vi "tm485_lightsheet.vi"() -> ()   [LabVIEW 2011]
panel:
  in  "Input Trigger Polarity":u32(ring)=1 items=["NEGATIVE"=1, "POSITIVE"=2]
  in  "Input Trigger Mode":u32(ring)=1 items=["INTERNAL"=1, "EXTERNAL EDGE"=2, "EXTERNAL LEVEL"=4, "SOFTWARE"=32, "FAST REPETITION"=64, "TDI"=128, "START"=512, "SYNC READOUT"=1024]
  in  "Internal Line Interval":dbl=9.74436e-06
  in  "Output Trigger Period":dbl=1e-05
  in  "Output Trigger Polarity":u32(ring)=1 items=["NEGATIVE"=1, "POSITIVE"=2]
  in  "Output Trigger Mode":u32(ring)=3 items=["LOW"=1, "GLOBAL EXPOSURE"=2, "PROGRAMMABLE"=3, "TRIGGER READY"=4, "HIGH"=5]
  in  "Readout Direction":u32(ring)=1 items=["FORWARD"=1, "BACKWARD"=2]
  in  "Pre Hsync Count":u32
  out "Image":u16[][](graph)
  out "Frames Per Second":dbl
  in  "Quit":bool
  out "Error Out":errorcluster {"code" format="%.0x"}
  # "This is just a simple example\nof how to setup a camera for\na Lightsheet application with\na Flash4.0 V2"
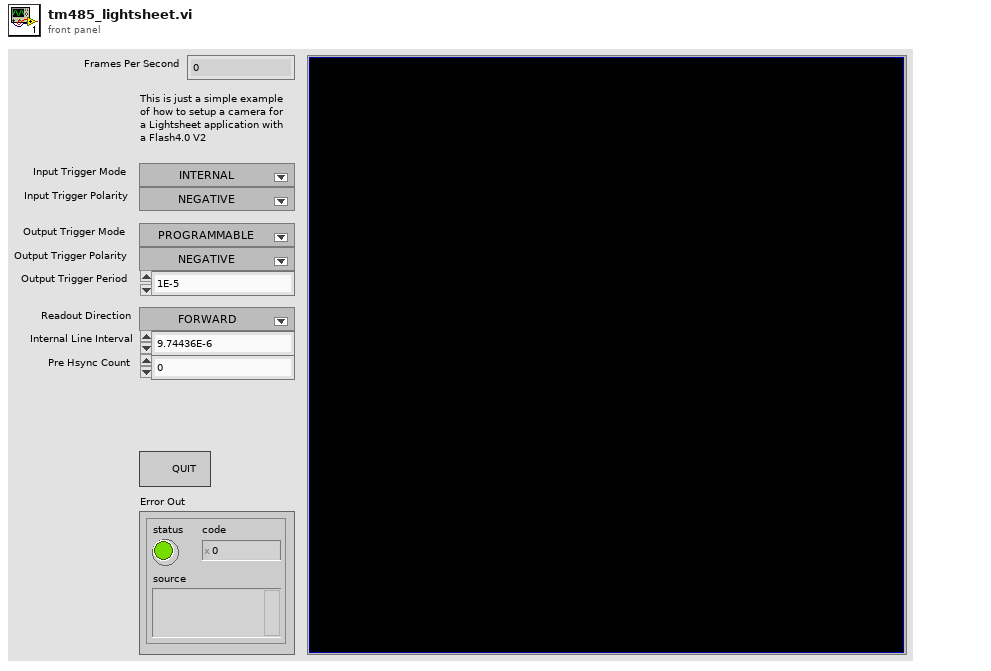
[diagram p1: front panel]
types:
  T1 = cluster{"Input Trigger Mode":u32, "Input Trigger Polarity":u32, "Times":u32, "Delay":dbl}
  T2 = cluster{"Output Trigger Mode":u32, "Output Trigger Polarity":u32}
  T3 = cluster{"Output Trigger Period":dbl, "Delay":dbl, "Source":u32}
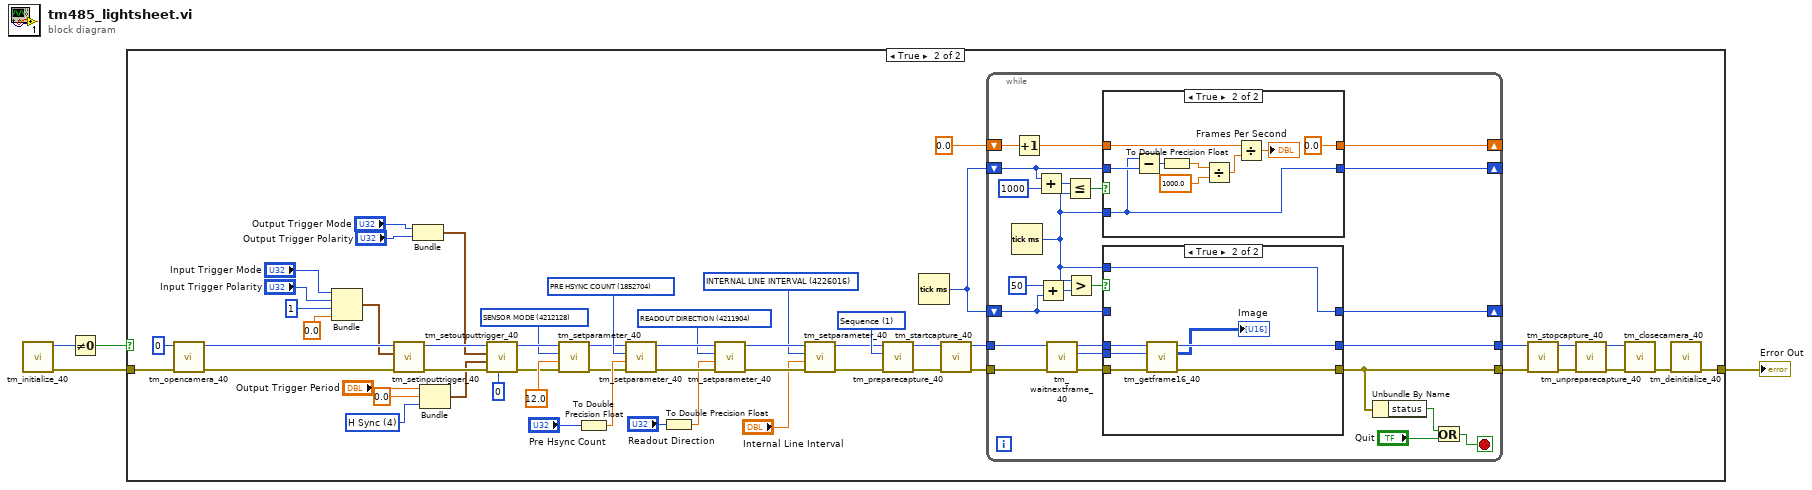
[diagram p0: block diagram]
diagram:
  n1 = call <userlib>:"tm_initialize_40.vi"() -> ("error out"=w1:errorcluster, "Number Of Cameras"=w2:u32)  [unwired: 8 in, 2 out]
  n2 = Not Equal To 0?(x=w2) -> (x != 0?=w4:bool)
  n3 = case shown="True" w4 {
    tunnel: w1 -> [w5 w59]
    tunnel: [w5 w56] -> w3
    frame False {
    }
    frame True {
      w8 = u32 4 items=["Exposure"=1, "Readout End"=2, "V Sync"=3, "H Sync"=4, "Trigger"=6] ("Source")
      w20 = u32 4226016 items=["SENSOR MODE"=4212128, "CCD MODE"=4212384, "READOUT MODE"=4211872, "ACTIVE VIEW INDEX"=4343136, "BITS PER CHANNEL"=4342976, "IMAGE PIXEL TYPE"=4343296, "BINNING"=4215968, "EXPOSURE TIME"=2049184, "CONTRAST GAIN"=3163312, "CONTRAST OFFSET"=3163328, "LIGHT MODE"=2114720, "SENSITIVITY"=2114992, "PHOTON IMAGING MODE"=2115200, "HIGH DYNAMIC RANGE MODE"=3163360, "WHITE BALANCE"=3163568, "TEMPERATURE"=2115232, "TEMPERATURE TARGET"=2115264, "SENSOR COOLER FAN"=2115296, "LINEBUNDLE HEIGHT"=4212192, "MECHANICAL SHUTTER"=2115488, "BACK FOCUS POSITION"=8422304, "TRIGGER CONNECTOR"=1066432, "TRIGGER SOURCE"=1066144, "OUTPUT TRIGGER SOURCE"=1852576, "TRIGGER GLOBAL EXPOSURE"=2049680, "FIRST TRIGGER BEHAVIOR"=2049696, "CHANNEL SYNC"=1852352, "READOUT DIRECTION"=4211904, "PRE HSYNC COUNT"=1852704, "INTERNAL LINE SPEED"=4226000, "INTERNAL LINE INTERVAL"=4226016] ("Parameter")
      w26 = u32 4212128 items=["SENSOR MODE"=4212128, "CCD MODE"=4212384, "READOUT MODE"=4211872, "ACTIVE VIEW INDEX"=4343136, "BITS PER CHANNEL"=4342976, "IMAGE PIXEL TYPE"=4343296, "BINNING"=4215968, "EXPOSURE TIME"=2049184, "CONTRAST GAIN"=3163312, "CONTRAST OFFSET"=3163328, "LIGHT MODE"=2114720, "SENSITIVITY"=2114992, "PHOTON IMAGING MODE"=2115200, "HIGH DYNAMIC RANGE MODE"=3163360, "WHITE BALANCE"=3163568, "TEMPERATURE"=2115232, "TEMPERATURE TARGET"=2115264, "SENSOR COOLER FAN"=2115296, "LINEBUNDLE HEIGHT"=4212192, "MECHANICAL SHUTTER"=2115488, "BACK FOCUS POSITION"=8422304, "TRIGGER CONNECTOR"=1066432, "TRIGGER SOURCE"=1066144, "OUTPUT TRIGGER SOURCE"=1852576, "TRIGGER GLOBAL EXPOSURE"=2049680, "FIRST TRIGGER BEHAVIOR"=2049696, "CHANNEL SYNC"=1852352, "READOUT DIRECTION"=4211904, "PRE HSYNC COUNT"=1852704, "INTERNAL LINE SPEED"=4191408, "INTERNAL LINE INTERVAL"=4191424] ("Parameter")
      w27 = u32 1852704 items=["SENSOR MODE"=4212128, "CCD MODE"=4212384, "READOUT MODE"=4211872, "ACTIVE VIEW INDEX"=4343136, "BITS PER CHANNEL"=4342976, "IMAGE PIXEL TYPE"=4343296, "BINNING"=4215968, "EXPOSURE TIME"=2049184, "CONTRAST GAIN"=3163312, "CONTRAST OFFSET"=3163328, "LIGHT MODE"=2114720, "SENSITIVITY"=2114992, "PHOTON IMAGING MODE"=2115200, "HIGH DYNAMIC RANGE MODE"=3163360, "WHITE BALANCE"=3163568, "TEMPERATURE"=2115232, "TEMPERATURE TARGET"=2115264, "SENSOR COOLER FAN"=2115296, "LINEBUNDLE HEIGHT"=4212192, "MECHANICAL SHUTTER"=2115488, "BACK FOCUS POSITION"=8422304, "TRIGGER CONNECTOR"=1066432, "TRIGGER SOURCE"=1066144, "OUTPUT TRIGGER SOURCE"=1852576, "TRIGGER GLOBAL EXPOSURE"=2049680, "FIRST TRIGGER BEHAVIOR"=2049696, "CHANNEL SYNC"=1852352, "READOUT DIRECTION"=4211904, "PRE HSYNC COUNT"=1852704, "INTERNAL LINE SPEED"=4191408, "INTERNAL LINE INTERVAL"=4191424] ("Parameter")
      w28 = u32 4211904 items=["SENSOR MODE"=4212128, "CCD MODE"=4212384, "READOUT MODE"=4211872, "ACTIVE VIEW INDEX"=4343136, "BITS PER CHANNEL"=4342976, "IMAGE PIXEL TYPE"=4343296, "BINNING"=4215968, "EXPOSURE TIME"=2049184, "CONTRAST GAIN"=3163312, "CONTRAST OFFSET"=3163328, "LIGHT MODE"=2114720, "SENSITIVITY"=2114992, "PHOTON IMAGING MODE"=2115200, "HIGH DYNAMIC RANGE MODE"=3163360, "WHITE BALANCE"=3163568, "TEMPERATURE"=2115232, "TEMPERATURE TARGET"=2115264, "SENSOR COOLER FAN"=2115296, "LINEBUNDLE HEIGHT"=4212192, "MECHANICAL SHUTTER"=2115488, "BACK FOCUS POSITION"=8422304, "TRIGGER CONNECTOR"=1066432, "TRIGGER SOURCE"=1066144, "OUTPUT TRIGGER SOURCE"=1852576, "TRIGGER GLOBAL EXPOSURE"=2049680, "FIRST TRIGGER BEHAVIOR"=2049696, "CHANNEL SYNC"=1852352, "READOUT DIRECTION"=4211904, "PRE HSYNC COUNT"=1852704, "INTERNAL LINE SPEED"=4191408, "INTERNAL LINE INTERVAL"=4191424] ("Parameter")
      w47 = 1 items=["Snap", "Sequence"] ("Capture mode")
      n4 = call <userlib>:"tm_opencamera_40.vi"("error in (no error)"=w59, "Camera Index"=u32 0) -> ("error out"=w31:errorcluster, "Handle out"=w32:u32)  [unwired: 7 in, 1 out]
      n5 = Bundle("Input Trigger Mode"="Input Trigger Mode", "Input Trigger Polarity"="Input Trigger Polarity", "Times"=u32 1, "Delay"=0.0) -> (w19:T1)  [unwired: 1 in]
      n6 = call <userlib>:"tm_setinputtrigger_40.vi"("error in (no error)"=w31, "Parameters"=w19, "Handle in"=w32) -> ("error out"=w34:errorcluster, "Handle out"=w33:u32)  [unwired: 7 in]
      n7 = Bundle("Output Trigger Mode"="Output Trigger Mode", "Output Trigger Polarity"="Output Trigger Polarity") -> (w12:T2)  [unwired: 1 in]
      n8 = Bundle("Output Trigger Period"="Output Trigger Period", "Delay"=0.0, "Source"=w8) -> (w11:T3)  [unwired: 1 in]
      n9 = call <userlib>:"tm_setoutputtrigger_40.vi"("Port"=0 ("Index"), "error in (no error)"=w34, "Programmable Options"=w11, "Type"=w12, "Handle in"=w33) -> ("error out"=w29:errorcluster, "Handle out"=w30:u32)  [unwired: 5 in]
      n10 = call <userlib>:"tm_setparameter_40.vi"("error in (no error)"=w29, "Value in"=12.0, "Parameter"=w26, "Handle in"=w30) -> ("error out"=w6:errorcluster, "Handle out"=w7:u32)  [unwired: 6 in]
      n11 = To Double Precision Float(number="Pre Hsync Count") -> (double precision float=w41:dbl)
      n12 = call <userlib>:"tm_setparameter_40.vi"("error in (no error)"=w6, "Value in"=w41, "Parameter"=w27, "Handle in"=w7) -> ("error out"=w39:errorcluster, "Handle out"=w38:u32)  [unwired: 6 in]
      n13 = To Double Precision Float(number="Readout Direction") -> (double precision float=w37:dbl)
      n14 = call <userlib>:"tm_setparameter_40.vi"("error in (no error)"=w39, "Value in"=w37, "Parameter"=w28, "Handle in"=w38) -> ("error out"=w24:errorcluster, "Handle out"=w25:u32)  [unwired: 6 in]
      n15 = call <userlib>:"tm_setparameter_40.vi"("error in (no error)"=w24, "Value in"="Internal Line Interval", "Parameter"=w20, "Handle in"=w25) -> ("error out"=w22:errorcluster, "Handle out"=w21:u32)  [unwired: 6 in]
      n16 = call <userlib>:"tm_preparecapture_40.vi"("error in (no error)"=w22, "Capture mode"=w47, "Handle in"=w21) -> ("error out"=w45:errorcluster, "Handle out"=w46:u32)  [unwired: 5 in, 2 out]
      n17 = Tick Count (ms)() -> (millisecond timer value=w43:u32)
      n18 = call <userlib>:"tm_startcapture_40.vi"("error in (no error)"=w45, "Handle in"=w46) -> ("error out"=w48:errorcluster, "Handle out"=w49:u32)  [unwired: 8 in]
      n19 = while {
        tunnel: [w62] -> w52
        tunnel: [w63] -> w53
        tunnel: w49 -> [w80]
        tunnel: w48 -> [w81]
        shift-right: [w78] -> _
        shift-left: w43 -> [w75]
        shift-right: [w79] -> _
        shift-left: 0.0 -> [w72]
        shift-right: [w61] -> _
        shift-left: w43 -> [w64]
        stop <- w60 stop-if-true
        n20 = Tick Count (ms)() -> (millisecond timer value=w65:u32)
        n21 = Increment(x=w72) -> (x+1=w73:dbl)
        n22 = Add(x=w75, y=u32 1000) -> (x+y=w77:u32)
        n23 = Add(x=u32 50, y=w64) -> (x+y=w67:u32)
        n24 = call <userlib>:"tm_waitnextframe_40.vi"("error in (no error)"=w81, "Handle in"=w80) -> ("error out"=w70:errorcluster, "Frame Index"=w69:i32, "Handle out"=w71:u32)  [unwired: 6 in, 1 out]
        n25 = Less Or Equal?(x=w77, y=w65) -> (x <= y?=w74:bool)
        n26 = Greater?(x=w65, y=w67) -> (0:w66:bool)
        n27 = case shown="True" w74 {
          tunnel: w75 -> [w95 w98]
          tunnel: [w95 w96] -> w78
          tunnel: w73 -> [w94 w102]
          tunnel: w65 -> [_ w96]
          tunnel: [w94 0.0] -> w79
          frame False {
          }
          frame True {
            n28 = Subtract(x=w96, y=w98) -> (x-y=w97:u32)
            n29 = To Double Precision Float(number=w97) -> (double precision float=w104:dbl)
            n30 = Divide(x=w104, y=1000.0) -> (x/y=w101:dbl)
            n31 = Divide(x=w102, y=w101) -> (x/y=→"Frames Per Second":dbl)
          }
        }
        n32 = case shown="True" w66 {
          tunnel: w71 -> [w86 w93]
          tunnel: w70 -> [w85 w92]
          tunnel: w69 -> [_ w91]
          tunnel: w64 -> [w84 _]
          tunnel: w65 -> [_ w90]
          tunnel: [w86 w88] -> w62
          tunnel: [w85 w89] -> w63
          tunnel: [w84 w90] -> w61
          frame False {
          }
          frame True {
            n33 = call <userlib>:"tm_getframe16_40.vi"("error in (no error)"=w92, "Frame Index"=w91, "Handle in"=w93) -> ("error out"=w89:errorcluster, "Data"=→"Image":u16[][], "Handle out"=w88:u32)  [unwired: 5 in, 1 out]
          }
        }
        n34 = Unbundle By Name(w63) -> ("status"=w83:bool)
        n35 = Or(x=w83, y="Quit") -> (x .or. y?=w60:bool)
      }
      n36 = call <userlib>:"tm_stopcapture_40.vi"("error in (no error)"=w53, "Handle in"=w52) -> ("error out"=w50:errorcluster, "Handle out"=w51:u32)  [unwired: 8 in]
      n37 = call <userlib>:"tm_unpreparecapture_40.vi"("error in (no error)"=w50, "Handle in"=w51) -> ("error out"=w55:errorcluster, "Handle out"=w54:u32)  [unwired: 8 in]
      n38 = call <userlib>:"tm_closecamera_40.vi"("error in (no error)"=w55, "Handle in"=w54) -> ("error out"=w57:errorcluster)  [unwired: 9 in]
      n39 = call <userlib>:"tm_deinitialize_40.vi"("error in (no error)"=w57) -> ("error out"=w56:errorcluster)  [unwired: 10 in]
    }
  }
  "Error Out" <- w3
